vi "pump calibration.vi"(4 "pump ID":u8, 6 "pump cal command":T3=enum."Save default values", 8 "STAMP intercept":dbl, 9 "STAMP slope":dbl=2.52, 10 "flow rate":dbl[unit], 11 "Pump Calibration in":T1={"target 1"=0.0, "target 2"=0.0, "measured 1"=1e-06, "measured 2"=1e-06}) -> (0 "STAMP intercept out":dbl, 1 "STAMP slope out":dbl=2.52, 2 "modified flow rate":dbl[unit], 3 "Pump Calibration out":T1)   [LabVIEW 2019]
uses:
  calibration values.ctl
  calibration commands.ctl
  Process Controller 3.0/Calibration and Function folders.ctl
  <vilib>/Utility/config.llb/Write Key (Double).vi
  <vilib>/Utility/config.llb/Read Key (Double).vi
  <vilib>/Utility/config.llb/NI_LVConfig.lvlib
panel:
  out "Selected Folder":path
  in  "pump calibrations default":T2(array[cluster])=[{"Pump Calibration"={"target 1"=0.0, "target 2"=1e-06, "measured 1"=0.0, "measured 2"=1e-06}, "STAMP slope"=1.0, "STAMP intercept"=0.0}, {"Pump Calibration"={"target 1"=0.0, "target 2"=1e-06, "measured 1"=0.0, "measured 2"=0.0}, "STAMP slope"=1.0, "STAMP intercept"=0.0}, {"Pump Calibration"={"target 1"=0.0, "target 2"=1e-06, "measured 1"=0.0, "measured 2"=0.0}, "STAMP slope"=1.0, "STAMP intercept"=0.0}, {"Pump Calibration"={"target 1"=0.0, "target 2"=1e-06, "measured 1"=0.0, "measured 2"=0.0}, "STAMP slope"=1.0, "STAMP intercept"=0.0}, {"Pump Calibration"={"target 1"=0.0, "target 2"=1e-06, "measured 1"=0.0, "measured 2"=0.0}, "STAMP slope"=1.0, "STAMP intercept"=0.0}, {"Pump Calibration"={"target 1"=0.0, "target 2"=1e-06, "measured 1"=0.0, "measured 2"=0.0}, "STAMP slope"=1.0, "STAMP intercept"=0.0}]
  out "pump calibrations":T2(array[cluster])
  in  "Pump Calibration default":T1={"target 1"=0.0, "target 2"=1e-06, "measured 1"=0.0, "measured 2"=1e-06}
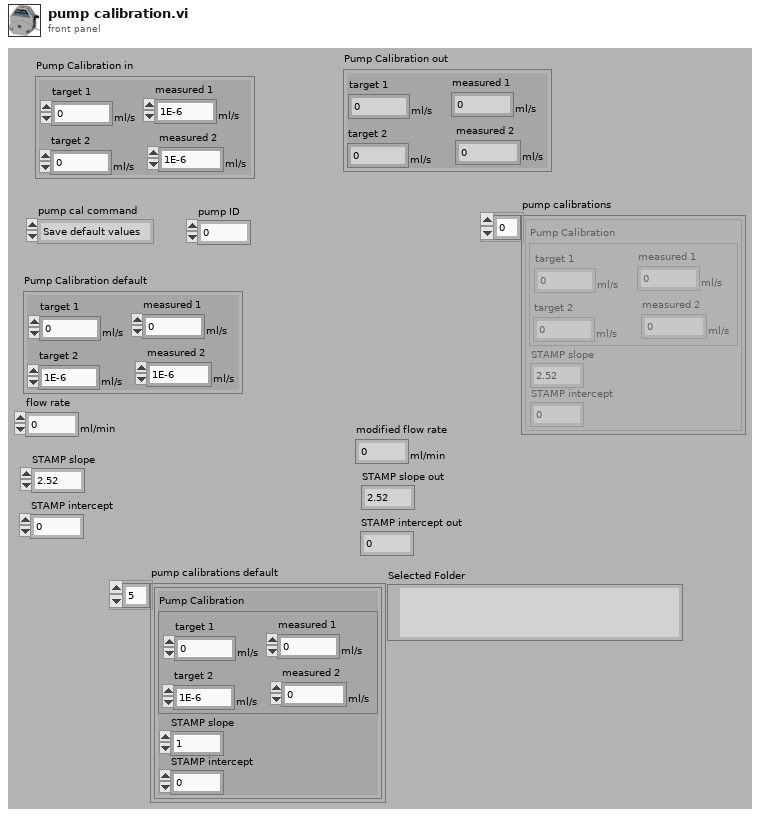
[diagram p1: front panel]
types:
  T1 = typedef "calibration values.ctl" = cluster{"target 1":dbl[unit], "target 2":dbl[unit], "measured 1":dbl[unit], "measured 2":dbl[unit]}
  T2 = cluster{"Pump Calibration":T1, "STAMP slope":dbl, "STAMP intercept":dbl}[]
  T3 = typedef "calibration commands.ctl" = enum16{"Get ini Path", "Save default values", "Save new calibration", "Read calibration", "Apply calibration", "Read STAMP mb", "Write STAMP mb"}
  T4 = typedef "Calibration and Function folders.ctl" = enum16{"Sensors", "Functions", "Config File", "PublicAppFolder", "New ini File", "Set Config File", "Delete ini File"}
  T5 = typedef "NI_LVConfig.lvlib/Config Data RefNum.ctl" = refnum<k1>
  T6 = cluster{"Pump Calibration":T1, "STAMP slope":dbl, "STAMP intercept":dbl}
  T7 = cluster{"[0]":dbl[unit], "[1]":dbl[unit], "[2]":dbl[unit], "[3]":dbl[unit]}
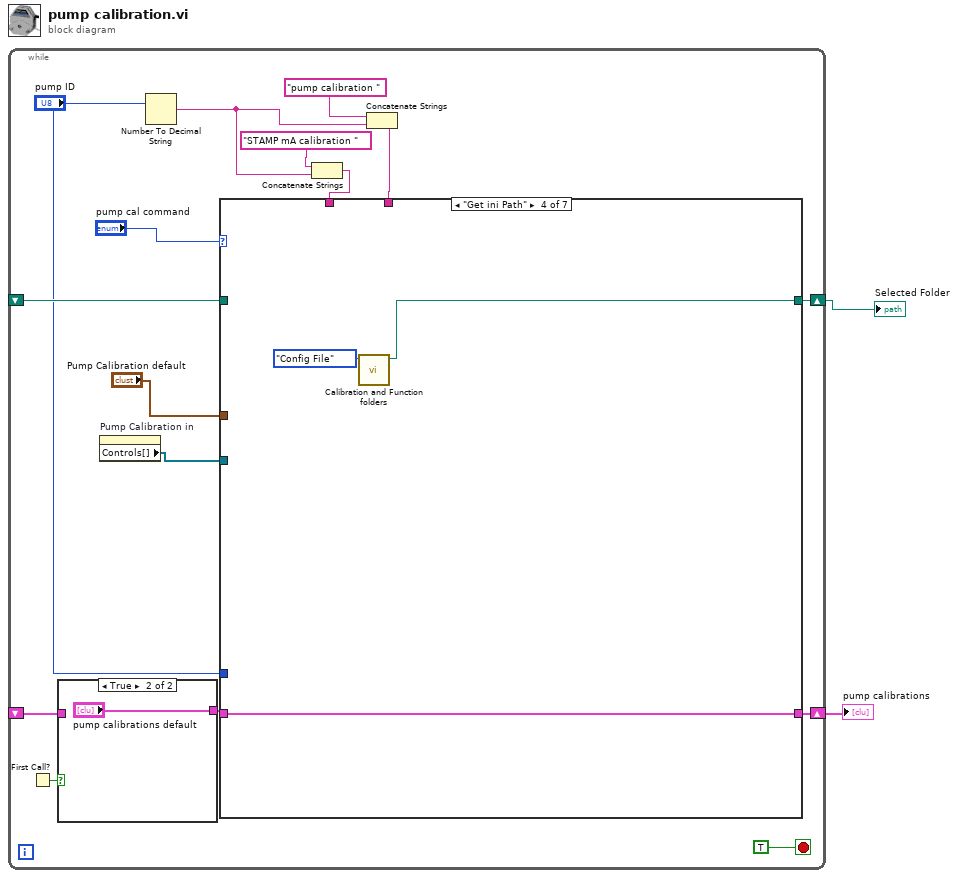
[diagram p0: block diagram]
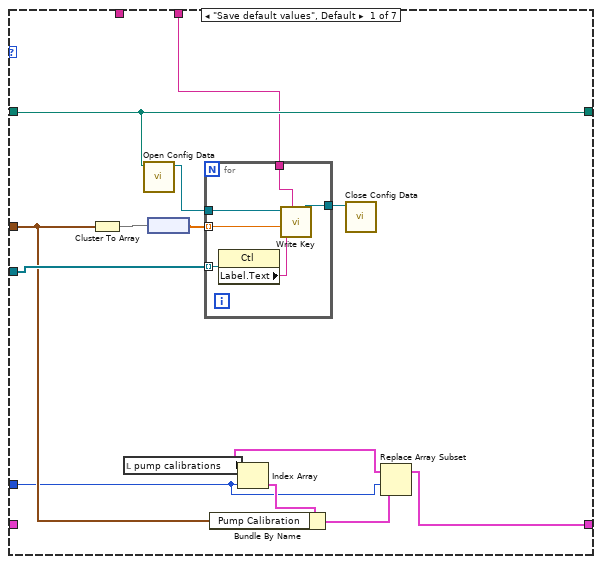
[diagram p3: hidden frame]
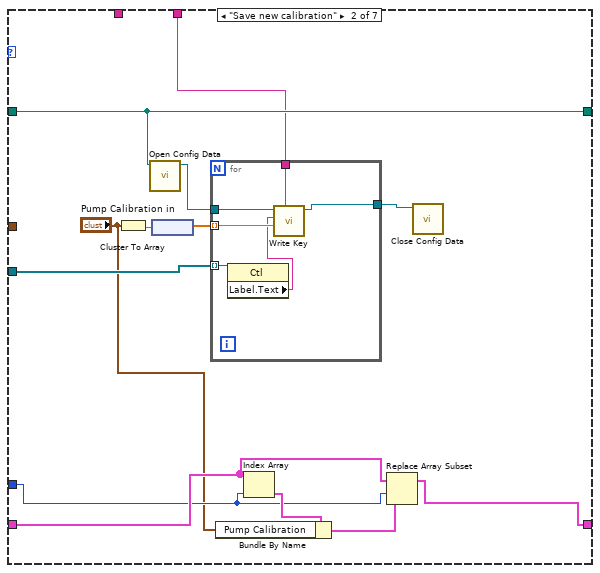
[diagram p4: hidden frame]
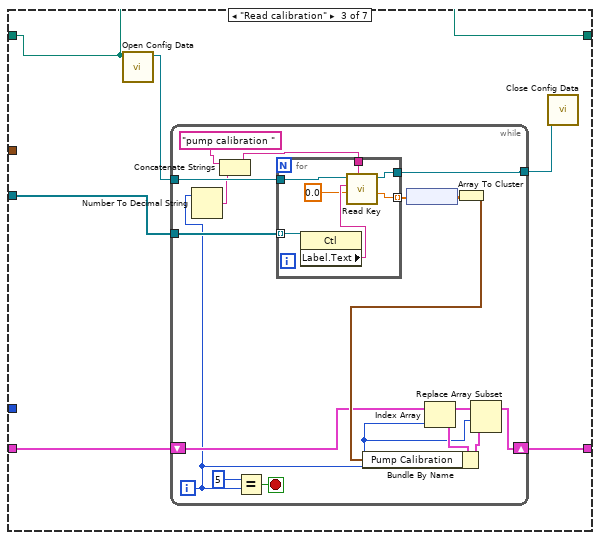
[diagram p5: hidden frame]
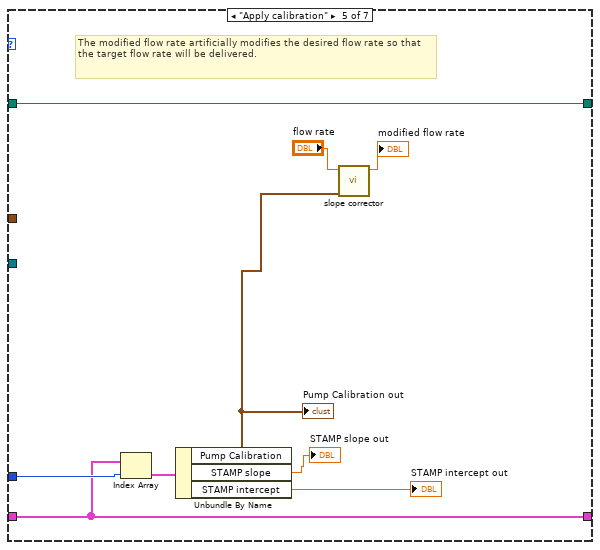
[diagram p6: hidden frame]
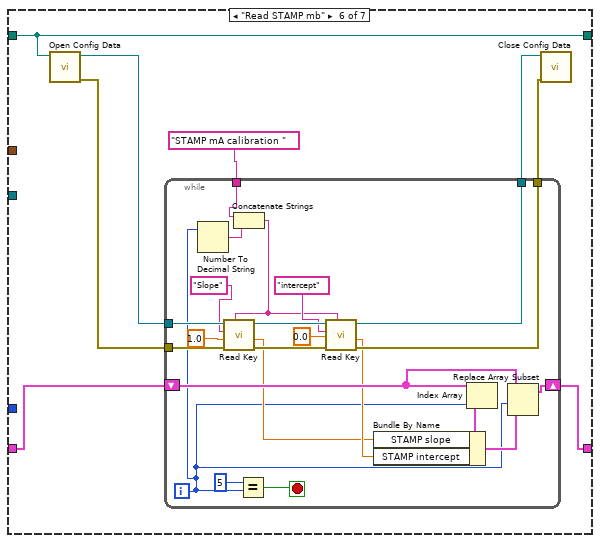
[diagram p7: hidden frame]
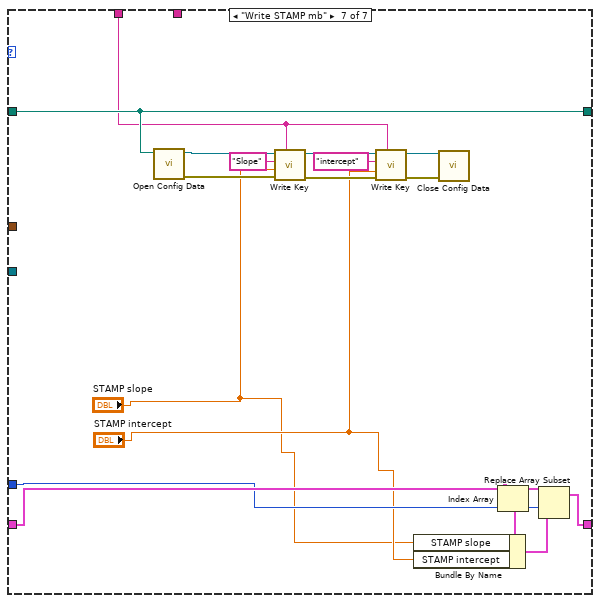
[diagram p8: hidden frame]
diagram:
  n1 = while {
    shift-right: [w15] -> w1
    shift-left: _ -> [w17]
    shift-right: [w6] -> w2
    shift-left: _ -> [w4]
    stop <- TRUE stop-if-true
    n2 = First Call?() -> (First Call?: T/F=w5:bool)
    n3 = case shown="True" w5 {
      tunnel: w4 -> [w19 _]
      tunnel: [w19 "pump calibrations default"] -> w3
      frame False {
      }
      frame True {
      }
    }
    n4 = property on="Pump Calibration in" class="Clust (strict)"() -> ("Controls[]"=w16:refnum<vi>[])  [unwired: 2 in, 2 out]
    n5 = Number To Decimal String(number="pump ID") -> (decimal integer string=w9:string)  [unwired: 1 in]
    n6 = Concatenate Strings("STAMP mA calibration " ("section"), w9) -> (w8:string)
    n7 = Concatenate Strings("pump calibration " ("section"), w9) -> (w11:string)
    n8 = case shown="\"Get ini Path\"" "pump cal command" {
      tunnel: w17 -> [w30 w50 w61 _ w99 w107 w146]
      tunnel: w16 -> [w29 w49 w62 _ _ _ _]
      tunnel: [w30 w50 w61 w88 w99 w107 w146] -> w15
      tunnel: w8 -> [_ _ _ _ _ _ w137]
      tunnel: w11 -> [w27 w46 _ _ _ _ _]
      tunnel: "Pump Calibration default" -> [w25 _ _ _ _ _ _]
      tunnel: "pump ID" -> [w23 w41 _ _ w96 _ w132]
      tunnel: [w21 w43 w59 w90 w95 w101 w134] -> w6
      tunnel: w3 -> [_ w42 w60 w90 w95 w102 w133]
      frame "Save default values", Default {
        n9 = Cluster To Array(cluster=w25) -> (array=w32:dbl[unit][])
        n10 = local read "pump calibrations"() -> (w24:T2)
        n11 = call <vilib>:"Open Config Data.vi"("configuration file path"=w30) -> ("refnum"=w33:T5)  [unwired: 8 in, 2 out]
        n12 = node(w32) -> (w28:dbl[])
        n13 = for {
          tunnel: w33 -> [w39]
          tunnel: w28 -> [w38] mode=indexing
          tunnel: w29 -> [w37] mode=indexing
          tunnel: w27 -> [w35]
          tunnel: [w34] -> w31
          n14 = property class="Ctl"(reference=w37) -> ("Label.Text"=w36:string)  [unwired: 1 in, 2 out]
          n15 = call-poly <vilib>:"Write Key.vi"("section"=w35, "value"=w38, "key"=w36, "refnum"=w39) -> ("refnum out"=w34:T5)  [unwired: 5 in, 2 out]
        }
        n16 = Index Array(array=w24, index=w23) -> (element=w26:T6)
        n17 = Bundle By Name(cluster=w26, "Pump Calibration"=w25) -> (w22:T6)
        n18 = call <vilib>:"Close Config Data.vi"("refnum"=w31) -> ()  [unwired: 9 in, 2 out]
        n19 = Replace Array Subset(array=w24, new element=w22, index=w23) -> (w21:T2)
      }
      frame "Save new calibration" {
        n20 = Cluster To Array(cluster="Pump Calibration in") -> (array=w47:dbl[unit][])
        n21 = call <vilib>:"Open Config Data.vi"("configuration file path"=w50) -> ("refnum"=w52:T5)  [unwired: 8 in, 2 out]
        n22 = node(w47) -> (w48:dbl[])
        n23 = for {
          tunnel: w52 -> [w58]
          tunnel: w48 -> [w57] mode=indexing
          tunnel: w49 -> [w56] mode=indexing
          tunnel: w46 -> [w54]
          tunnel: [w53] -> w51
          n24 = property class="Ctl"(reference=w56) -> ("Label.Text"=w55:string)  [unwired: 1 in, 2 out]
          n25 = call-poly <vilib>:"Write Key.vi"("section"=w54, "value"=w57, "key"=w55, "refnum"=w58) -> ("refnum out"=w53:T5)  [unwired: 5 in, 2 out]
        }
        n26 = Index Array(array=w42, index=w41) -> (element=w45:T6)
        n27 = Bundle By Name(cluster=w45, "Pump Calibration"="Pump Calibration in") -> (w44:T6)
        n28 = Replace Array Subset(array=w42, new element=w44, index=w41) -> (w43:T2)
        n29 = call <vilib>:"Close Config Data.vi"("refnum"=w51) -> ()  [unwired: 9 in, 2 out]
      }
      frame "Read calibration" {
        n30 = call <vilib>:"Open Config Data.vi"("configuration file path"=w61) -> ("refnum"=w64:T5)  [unwired: 8 in, 2 out]
        n31 = while {
          tunnel: w64 -> [w80]
          tunnel: [w79] -> w63
          tunnel: w62 -> [w77]
          shift-right: [w71] -> w59
          shift-left: w60 -> [w72]
          i -> [w67]
          stop <- w65 stop-if-true
          n32 = Number To Decimal String(number=w67) -> (decimal integer string=w69:string)  [unwired: 1 in]
          n33 = Concatenate Strings("pump calibration " ("section"), w69) -> (w68:string)
          n34 = Equal?(x=5, y=w67) -> (x = y?=w65:bool)
          n35 = for {
            tunnel: w80 -> [w87]
            tunnel: w77 -> [w86] mode=indexing
            tunnel: w68 -> [w84]
            tunnel: [w83] -> w79
            tunnel: [w81] -> w78 mode=indexing
            n36 = property class="Ctl"(reference=w86) -> ("Label.Text"=w85:string)  [unwired: 1 in, 2 out]
            n37 = call-poly <vilib>:"Read Key.vi"("section"=w84, "default value"=0.0 ("target 1"), "key"=w85, "refnum"=w87) -> ("value"=w81:dbl, "refnum out"=w83:T5)  [unwired: 4 in, 2 out]
          }
          n38 = node(w78) -> (w76:dbl[unit][])
          n39 = Index Array(array=w72, index=w67) -> (element=w75:T6)
          n40 = Array To Cluster(array=w76) -> (cluster=w73:T7)
          n41 = Bundle By Name(cluster=w75, "Pump Calibration"=w73) -> (w74:T6)
          n42 = Replace Array Subset(array=w72, new element=w74, index=w67) -> (w71:T2)
        }
        n43 = call <vilib>:"Close Config Data.vi"("refnum"=w63) -> ()  [unwired: 9 in, 2 out]
      }
      frame "Get ini Path" {
        n44 = call "Calibration and Function folders.vi"("Folder"=Calibration_and_Function_folders."Config File") -> ("Selected Folder"=w88:path)  [unwired: 9 in, 1 out]
      }
      frame "Apply calibration" {
        # "The modified flow rate artificially modifies the desired flow rate so that the target flow rate will be delivered."
        n45 = Index Array(array=w95, index=w96) -> (element=w94:T6)
        n46 = Unbundle By Name(w94) -> ("Pump Calibration"=w91:T1, "STAMP slope"=→"STAMP slope out":dbl, "STAMP intercept"=→"STAMP intercept out":dbl)
        "Pump Calibration out" <- w91
        n47 = call "slope corrector.vi"("Pump Calibration"=w91, "flow rate"="flow rate") -> ("modified flow rate"=→"modified flow rate":dbl[unit])  [unwired: 9 in]
      }
      frame "Read STAMP mb" {
        n48 = call <vilib>:"Open Config Data.vi"("configuration file path"=w107) -> ("error out"=w104:errorcluster, "refnum"=w106:T5)  [unwired: 8 in, 1 out]
        n49 = while {
          tunnel: w106 -> [w129]
          tunnel: [w127] -> w105
          tunnel: w104 -> [w126]
          tunnel: [w124] -> w103
          shift-right: [w115] -> w101
          shift-left: w102 -> [w118]
          tunnel: "STAMP mA calibration " ("section") -> [w112]
          i -> [w110]
          stop <- w108 stop-if-true
          n50 = Number To Decimal String(number=w110) -> (decimal integer string=w111:string)  [unwired: 1 in]
          n51 = Concatenate Strings(w112, w111) -> (w113:string)
          n52 = call-poly <vilib>:"Read Key.vi"("section"=w113, "error in (no error)"=w126, "default value"=1.0 ("STAMP slope"), "key"="Slope", "refnum"=w129) -> ("error out"=w125:errorcluster, "value"=w116:dbl, "refnum out"=w128:T5)  [unwired: 3 in, 1 out]
          n53 = Equal?(x=5, y=w110) -> (x = y?=w108:bool)
          n54 = call-poly <vilib>:"Read Key.vi"("section"=w113, "error in (no error)"=w125, "default value"=0.0 ("STAMP intercept"), "key"="intercept", "refnum"=w128) -> ("error out"=w124:errorcluster, "value"=w117:dbl, "refnum out"=w127:T5)  [unwired: 3 in, 1 out]
          n55 = Index Array(array=w118, index=w110) -> (element=w120:T6)
          n56 = Bundle By Name(cluster=w120, "STAMP slope"=w116, "STAMP intercept"=w117) -> (w119:T6)
          n57 = Replace Array Subset(array=w118, new element=w119, index=w110) -> (w115:T2)
        }
        n58 = call <vilib>:"Close Config Data.vi"("error in (no error)"=w103, "refnum"=w105) -> ()  [unwired: 8 in, 2 out]
      }
      frame "Write STAMP mb" {
        n59 = call <vilib>:"Open Config Data.vi"("configuration file path"=w146) -> ("error out"=w140:errorcluster, "refnum"=w145:T5)  [unwired: 8 in, 1 out]
        n60 = call-poly <vilib>:"Write Key.vi"("section"=w137, "error in (no error)"=w140, "value"="STAMP slope", "key"="Slope", "refnum"=w145) -> ("error out"=w139:errorcluster, "refnum out"=w144:T5)  [unwired: 4 in, 1 out]
        n61 = call-poly <vilib>:"Write Key.vi"("section"=w137, "error in (no error)"=w139, "value"="STAMP intercept", "key"="intercept", "refnum"=w144) -> ("error out"=w138:errorcluster, "refnum out"=w143:T5)  [unwired: 4 in, 1 out]
        n62 = call <vilib>:"Close Config Data.vi"("error in (no error)"=w138, "refnum"=w143) -> ()  [unwired: 8 in, 2 out]
        n63 = Index Array(array=w133, index=w132) -> (element=w136:T6)
        n64 = Bundle By Name(cluster=w136, "STAMP slope"="STAMP slope", "STAMP intercept"="STAMP intercept") -> (w135:T6)
        n65 = Replace Array Subset(array=w133, new element=w135, index=w132) -> (w134:T2)
      }
    }
  }
  "pump calibrations" <- w2
  "Selected Folder" <- w1
